vi "Reference Imaging Source.vi"() -> ()   [LabVIEW 2014]
uses:
  <vilib>/userdefined/High Color/IMAQdx.ctl
  <vilib>/vision/driver/IMAQdx.llb/IMAQdx Buffer Number Mode.ctl
  <vilib>/vision/driver/NI_Vision_Acquisition_Software.lvlib
  <resource>/objmgr/imaqdx.rc
panel:
  out "Ref Path":path
  out "Init Message":string
  out "Device Serial Number":string
  out "Success?":bool
  out "error out  - closing camera":errorcluster
  out "Message":string
  out "Warning":bool
  in  "Overwrite?":bool
  in  "Exposure Time":dbl=1.0 min=5e-06 max=5.0 step=1e-05 format="%#_8f"
  out "Buffer Number Out":u32
  in  "Nom Ref":string="ref"
  in  "File Path (for Snap! function)":path
  in  "snap":bool
  in  "Gain (dB)":i64=18 min=34 max=255 step=1
  in  "File to ref":bool
  in  "Ref To File":bool
  in  "End Point 2":cluster{"X":i32, "Y":i32}
  in  "Start Point 2":cluster{"X":i32, "Y":i32}
  in  "End Point 1":cluster{"X":i32, "Y":i32}
  in  "Start Point 1":cluster{"X":i32, "Y":i32}
  out "error out":errorcluster
  in  "error in (no error)":errorcluster
  in  "Rectangle d'encardrement":T1
  in  "ref":bool
  out "Coordonnées":i32[](array[numeric])
  in  "stop":bool
  out "Image":T2(plugin-control)
  in  "Session":T3="cam0"
  # "Références Champs Proches/Champs Lointains"
  # "Utiliser outil OVALE pour effectuer la sélection"
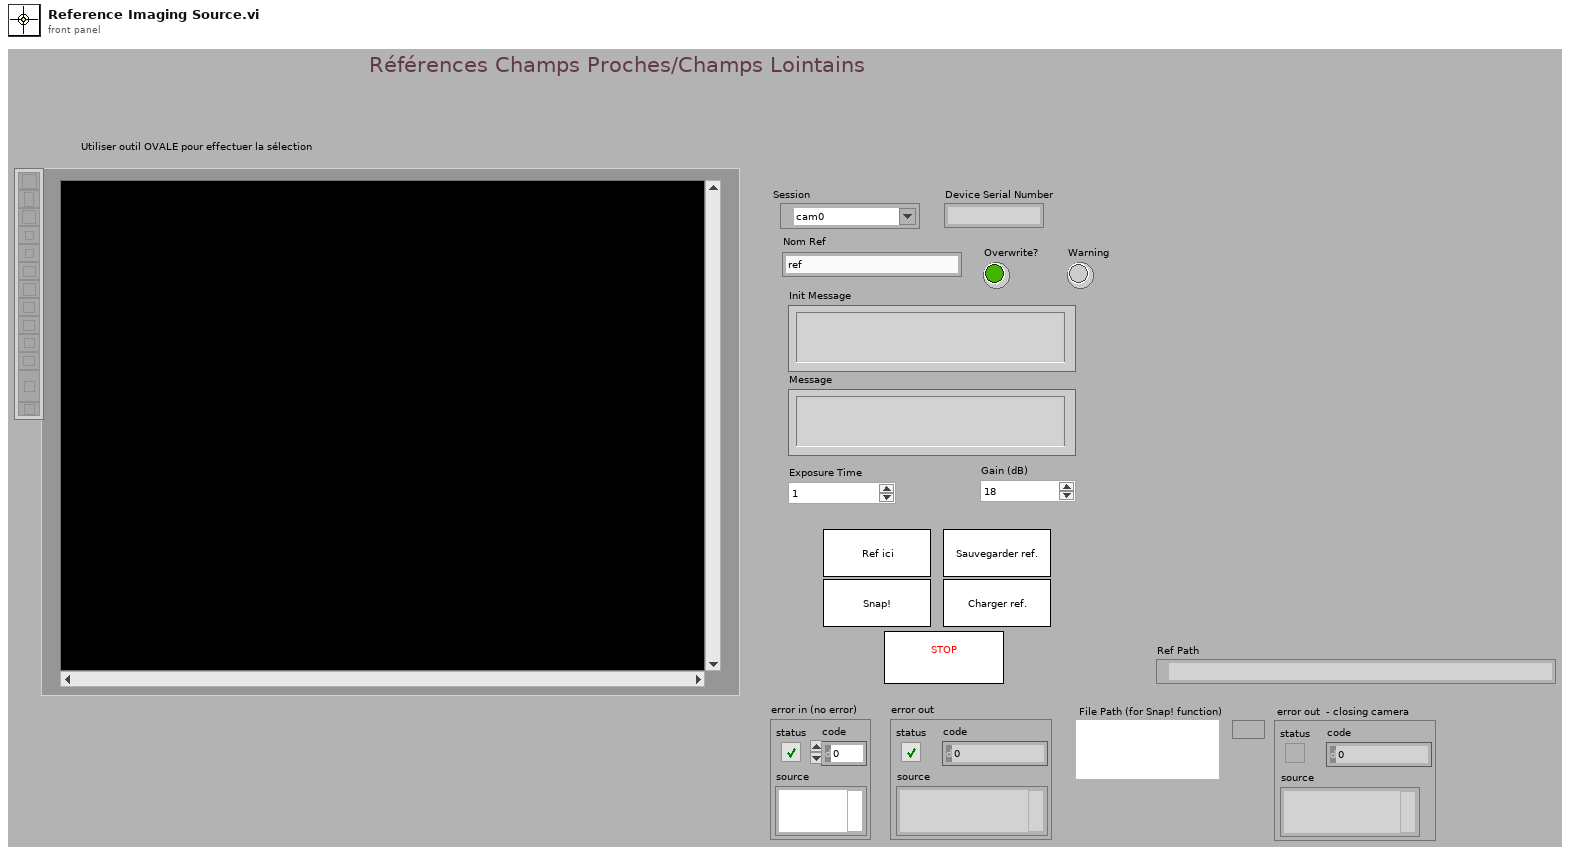
[diagram p1: front panel]
types:
  T1 = cluster{"Left":i32, "Top":i32, "Right":i32, "Bottom":i32}
  T2 = typedef "IMAQ Image.ctl" = refnum<image>
  T3 = typedef "IMAQdx.ctl" = refnum<k21>
  T4 = enum16{"open", "replace", "create", "open or create", "replace or create", "replace or create with confirmation"}
  T5 = typedef "NI_Vision_Acquisition_Software.lvlib/IMAQdx Buffer Number Mode.ctl" = enum32{"Next", "Last", "Buffer Number"}
  T6 = enum8{"Enabled", "Disabled", "Disabled and Grayed Out"}
  T7 = typedef "Image Type" = u32
  T8 = cluster{"Start Point 1":cluster{"X":i32, "Y":i32}, "End Point 1":cluster{"X":i32, "Y":i32}, "Start Point 2":cluster{"X":i32, "Y":i32}, "End Point 2":cluster{"X":i32, "Y":i32}}
  T9 = enum32{"invalid app kind", "Development System", "Run Time System", "Student Edition", "Embedded LabVIEW", "Evaluation", "Custom"}
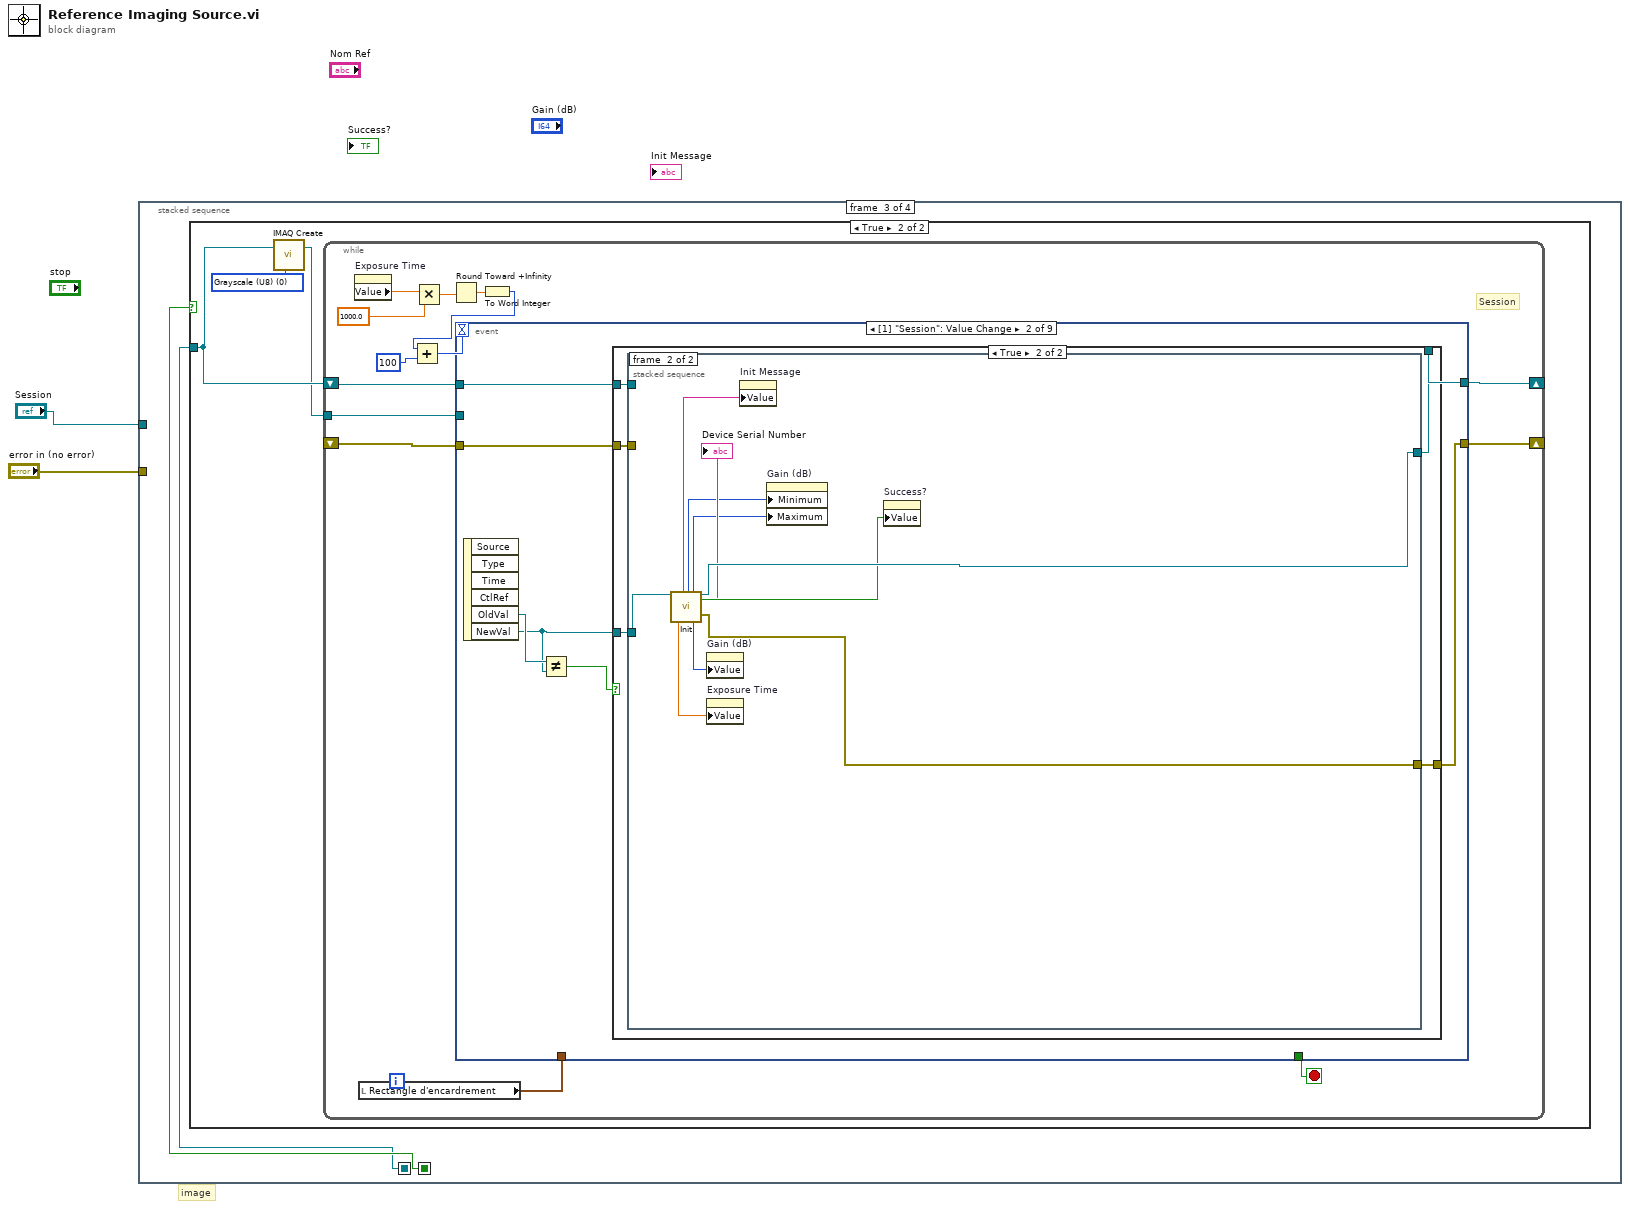
[diagram p0: block diagram]
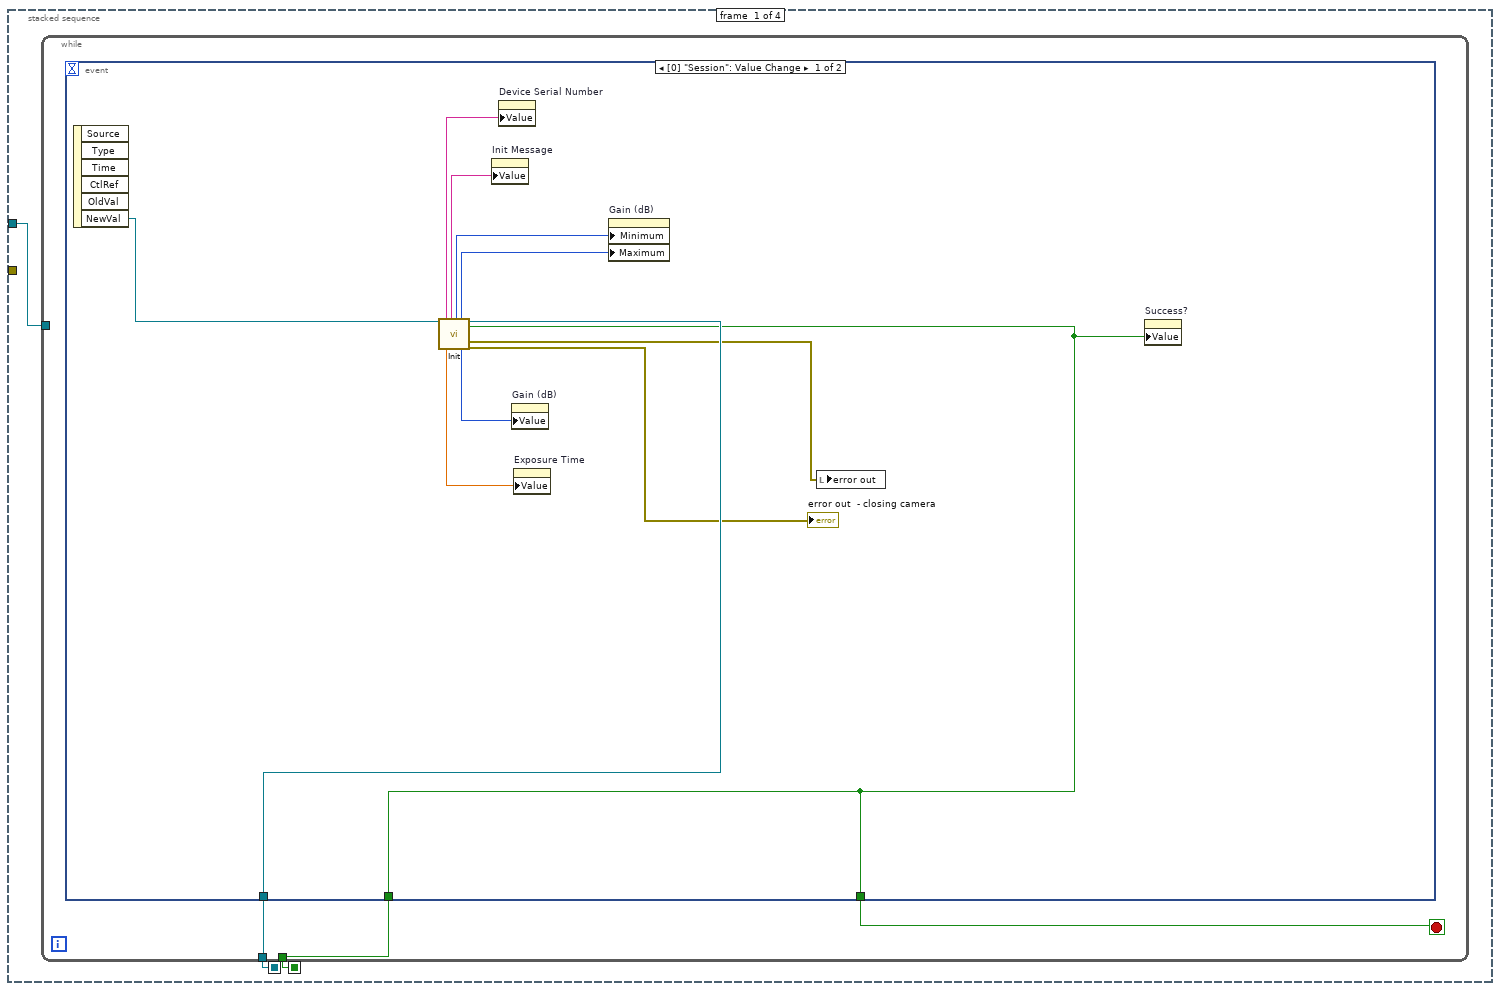
[diagram p2: hidden frame]
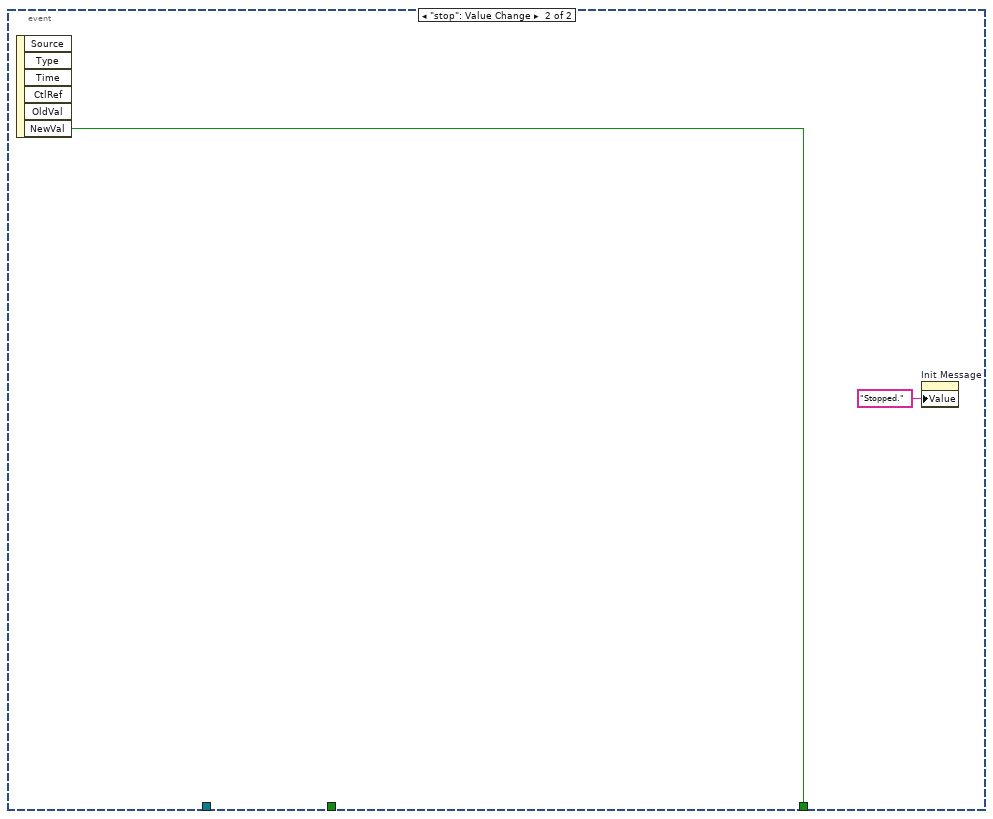
[diagram p3: hidden frame]
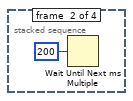
[diagram p4: hidden frame]
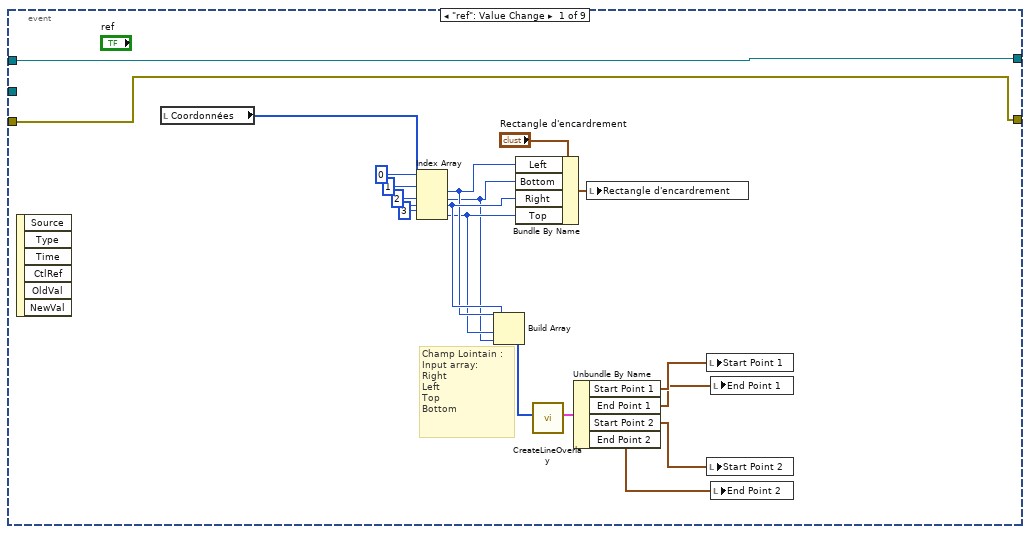
[diagram p6: hidden frame]
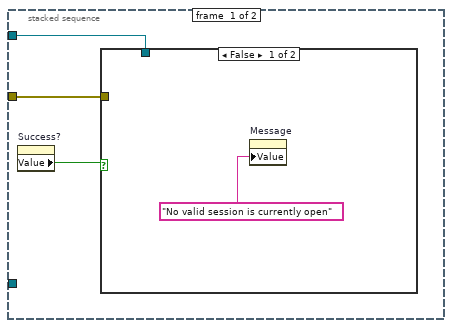
[diagram p8: hidden frame]
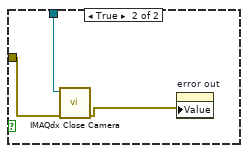
[diagram p9: hidden frame]
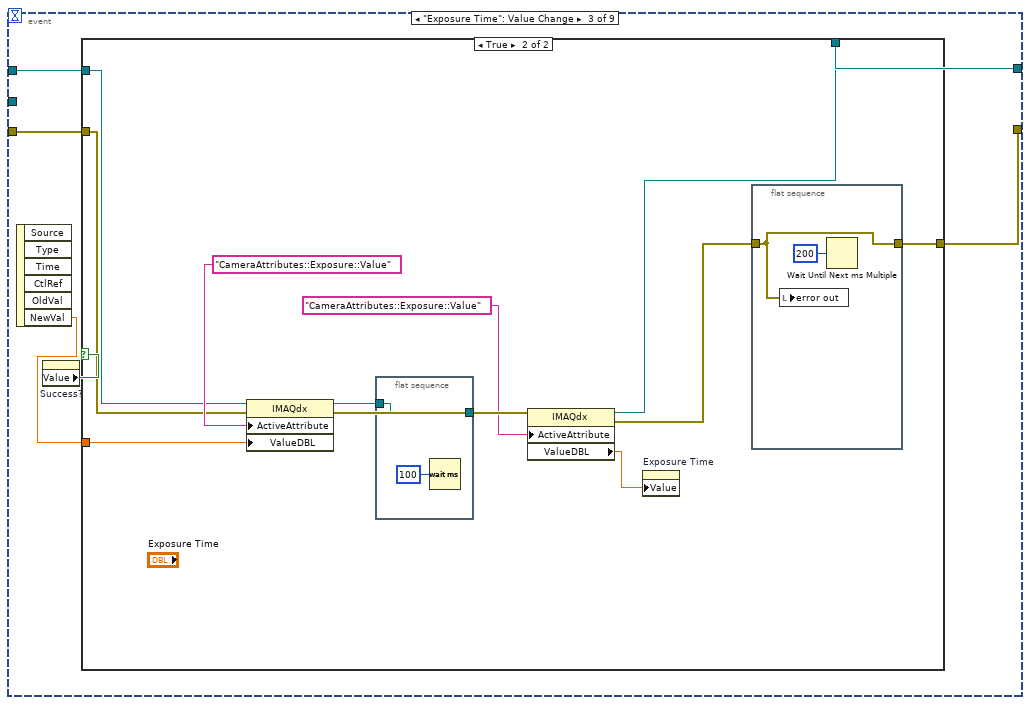
[diagram p10: hidden frame]
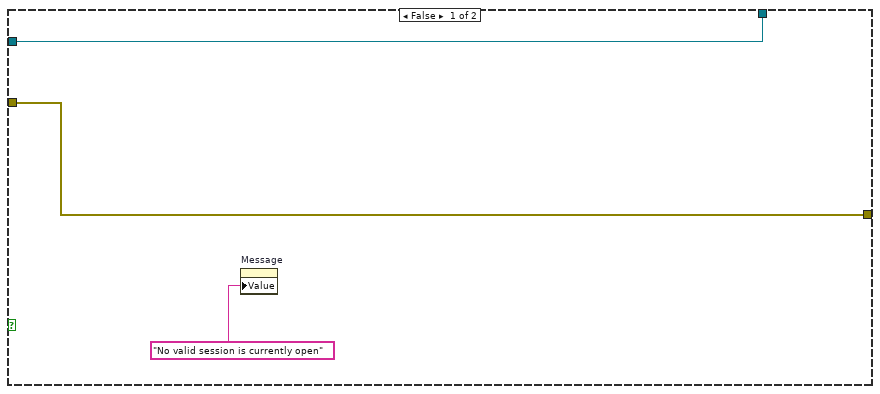
[diagram p11: hidden frame]
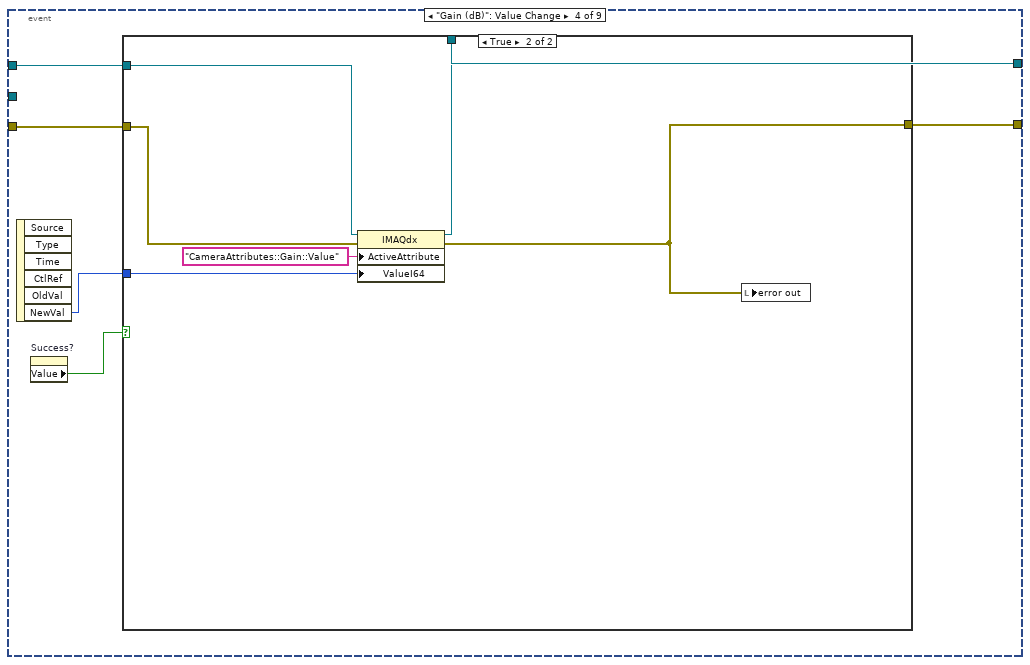
[diagram p12: hidden frame]
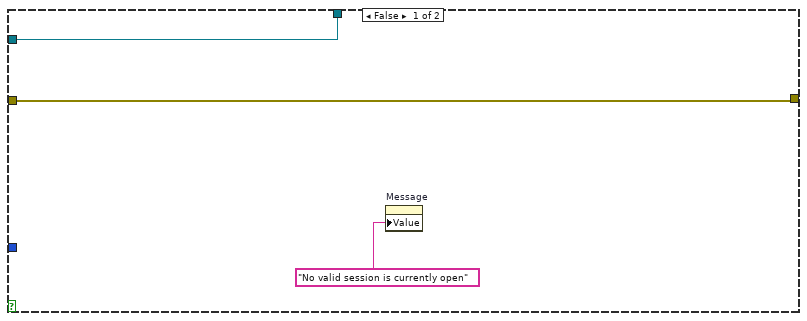
[diagram p13: hidden frame]
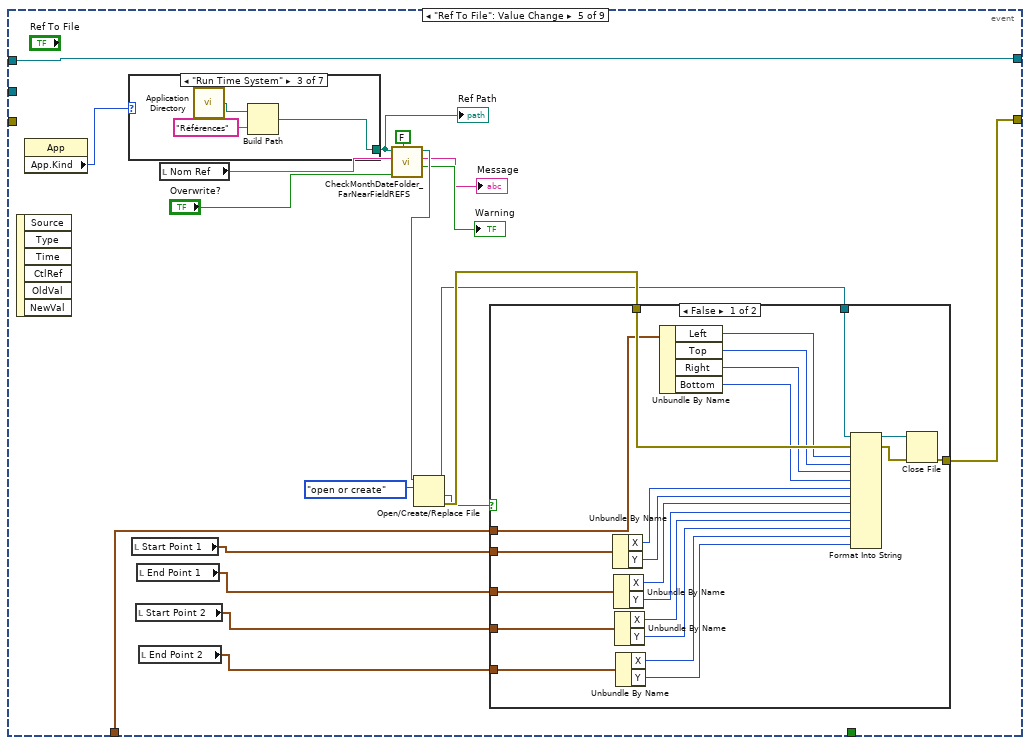
[diagram p14: hidden frame]
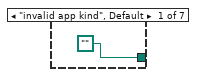
[diagram p15: hidden frame]
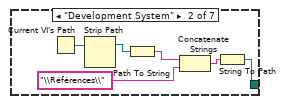
[diagram p16: hidden frame]
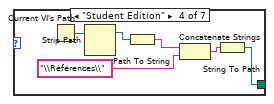
[diagram p17: hidden frame]
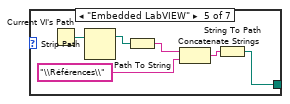
[diagram p18: hidden frame]
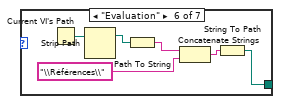
[diagram p19: hidden frame]
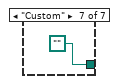
[diagram p20: hidden frame]
diagram:
  # "image"
  n1 = stacked-sequence {
    seq-local: [w4 _ _ _] -> [_ _ w23 _]
    seq-local: [w3 _ _ _] -> [_ _ w24 _]
    tunnel: "Session" -> [w5 _ _ _]
    tunnel: "error in (no error)" -> [_ _ _ _]
    frame #0 {
      n2 = while {
        tunnel: w5 -> [_]
        tunnel: [w7] -> w4
        tunnel: [w6] -> w3
        stop <- w8 stop-if-true
        n3 = event shown="[0] \"Session\": Value Change" {
          selector: _ -> [_ _]
          dyn-events: _ -> [_ _]
          timeout: _ -> [_ _]
          tunnel: [w11 w21] -> w8
          tunnel: [w19 _] -> w7
          tunnel: [w11 _] -> w6
          event Value Change {
            n4 = event-data() -> ("NewVal"=w18:T3)  [unwired: 1 in, 5 out]
            n5 = call "Init.vi"("Session"=w18) -> ("Device Serial Number"=w12:string, "Exposure Time - READ"=w16:dbl, "Message"=w13:string, "Gain Min"=w10:i64, "Gain Max"=w9:i64, "Gain - READ"=w17:i64, "IMAQdx Session OUT"=w19:T3, "Success?"=w11:bool, "error out"=w15:errorcluster, "error out  - closing camera"=→"error out  - closing camera":errorcluster)  [unwired: 9 in]
            n6 = property on="Init Message" class="Str"("Value"=w13) -> ()  [unwired: 2 in, 2 out]
            n7 = property on="Device Serial Number" class="Str"("Value"=w12) -> ()  [unwired: 2 in, 2 out]
            n8 = property on="Gain (dB)" class="DigNum (strict)"("Value"=w17) -> ()  [unwired: 2 in, 2 out]
            n9 = property on="Exposure Time" class="DigNum (strict)"("Value"=w16) -> ()  [unwired: 2 in, 2 out]
            n10 = property on="Gain (dB)" class="DigNum (strict)"("Minimum"=w10, "Maximum"=w9) -> ()  [unwired: 2 in, 2 out]
            n11 = local write "error out"(w15) -> ()
            n12 = property on="Success?" class="Bool (strict)"("Value"=w11) -> ()  [unwired: 2 in, 2 out]
          }
          event "stop": Value Change {
            n13 = event-data() -> ("NewVal"=w21:bool)  [unwired: 1 in, 5 out]
            n14 = property on="Init Message" class="Str"("Value"="Stopped." ("Init Message")) -> ()  [unwired: 2 in, 2 out]
          }
        }
      }
    }
    frame #1 {
      n15 = Wait Until Next ms Multiple(millisecond multiple=u32 200) -> ()  [unwired: 1 out]
    }
    frame #2 {
      n16 = case shown="True" w24 {
        tunnel: w23 -> [_ w26]
        frame False {
        }
        frame True {
          w27 = T7 0 items=["Grayscale (U8)", "Grayscale (I16)", "Grayscale (SGL)", "Complex (CSG)", "RGB (U32)", "HSL (U32)", "RGB (U64)", "Grayscale (U16)"] ("Image Type")
          n17 = call "IMAQ Create"("Image Name"=w26, "Image Type"=w27) -> ("New Image"=w25:T2)  [unwired: 2 in, 2 out]
          n18 = while {
            shift-right: [w39] -> _
            shift-left: _ -> [w40]
            shift-right: [w37] -> _
            shift-left: w26 -> [w38]
            tunnel: w25 -> [w28]
            stop <- w41 stop-if-true
            # "Session"
            n19 = property on="Exposure Time" class="DigNum (strict)"() -> ("Value"=w29:dbl)  [unwired: 2 in, 2 out]
            n20 = local read "Rectangle d'encardrement"() -> (w30:T1)
            n21 = Multiply(x=w29, y=1000.0) -> (x*y=w32:dbl)
            n22 = Round Toward +Infinity(x=w32) -> (ceil(x): smallest int >= x=w34:dbl)
            n23 = To Word Integer(number=w34) -> (16bit integer=w31:i16)
            n24 = Add(x=w31, y=i16 100) -> (x+y=w35:i16)
            n25 = event shown="[1] \"Session\": Value Change" {
              selector: _ -> [_ _ _ _ _ _ _ _ _]
              dyn-events: _ -> [_ _ _ _ _ _ _ _ _]
              timeout: w35 -> [_ _ _ _ _ _ _ _ _]
              tunnel: [_ _ _ _ _ _ _ w264 _] -> w41
              tunnel: w40 -> [w42 w67 w95 w122 _ w213 w248 w265 w278]
              tunnel: [w42 w65 w97 w119 w146 w208 w249 _ w277] -> w39
              tunnel: w38 -> [w43 w64 w96 w121 w134 w207 w247 w266 w276]
              tunnel: [w43 w66 w94 w120 w134 w207 w246 _ w275] -> w37
              tunnel: w30 -> [_ _ _ _ w145 _ _ _ _]
              tunnel: w28 -> [_ _ _ _ _ _ w245 _ w270]
              event "ref": Value Change {
                # "Champ Lointain :\nInput array:\nRight\nLeft\nTop\nBottom"
                n26 = event-data() -> ()  [unwired: 1 in, 6 out]
                n27 = local read "Coordonnées"() -> (w54:i32[])
                n28 = Index Array(array=w54, index #1=0 ("index"), index #2=1 ("index"), index #3=2 ("index"), index #4=3 ("index")) -> (element #1=w47:i32, element #2=w45:i32, element #3=w48:i32, element #4=w46:i32)
                n29 = Build Array(w48, w47, w46, w45) -> (w44:i32[])
                n30 = Bundle By Name(cluster="Rectangle d'encardrement", "Left"=w47, "Bottom"=w45, "Right"=w48, "Top"=w46) -> (w55:T1)
                n31 = call "CreateLineOverlay.vi"("Bounding rectangle"=w44) -> ("Lines"=w53:T8)  [unwired: 8 in, 1 out]
                n32 = Unbundle By Name(w53) -> ("Start Point 1"=w52:cluster{"X":i32, "Y":i32}, "End Point 1"=w51:cluster{"X":i32, "Y":i32}, "Start Point 2"=w50:cluster{"X":i32, "Y":i32}, "End Point 2"=w49:cluster{"X":i32, "Y":i32})
                n33 = local write "Rectangle d'encardrement"(w55) -> ()
                n34 = local write "Start Point 1"(w52) -> ()
                n35 = local write "Start Point 2"(w50) -> ()
                n36 = local write "End Point 1"(w51) -> ()
                n37 = local write "End Point 2"(w49) -> ()
              }
              event Value Change {
                n38 = event-data() -> ("OldVal"=w62:T3, "NewVal"=w61:T3)  [unwired: 1 in, 4 out]
                n39 = Not Equal?(x=w62, y=w61) -> (x != y?=w63:bool)
                n40 = case shown="True" w63 {
                  tunnel: w67 -> [w68 w74]
                  tunnel: w61 -> [w69 w73]
                  tunnel: [w69 w72] -> w66
                  tunnel: [w68 w71] -> w65
                  tunnel: w64 -> [_ w70]
                  frame False {
                  }
                  frame True {
                    n41 = stacked-sequence {
                      tunnel: w74 -> [w77 _]
                      tunnel: w73 -> [_ w91]
                      tunnel: [_ w88] -> w72
                      tunnel: [_ w86] -> w71
                      tunnel: w70 -> [w76 _]
                      frame #0 {
                        n42 = property on="Success?" class="Bool (strict)"() -> ("Value"=w75:bool)  [unwired: 2 in, 2 out]
                        n43 = case shown="False" w75 {
                          tunnel: w77 -> [_ w81]
                          tunnel: w76 -> [_ w79]
                          frame False {
                            n44 = property on="Message" class="Str"("Value"="No valid session is currently open" ("Message")) -> ()  [unwired: 2 in, 2 out]
                          }
                          frame True {
                            n45 = call <vilib>:"IMAQdx Close Camera.vi"("error in"=w81, "Session In"=w79) -> ("error out"=w80:errorcluster)  [unwired: 9 in]
                            n46 = property on="error out" class="Clust (strict)"("Value"=w80) -> ()  [unwired: 2 in, 2 out]
                          }
                        }
                      }
                      frame #1 {
                        n47 = call "Init.vi"("Session"=w91) -> ("Device Serial Number"=→"Device Serial Number":string, "Exposure Time - READ"=w89:dbl, "Message"=w84:string, "Gain Min"=w83:i64, "Gain Max"=w82:i64, "Gain - READ"=w90:i64, "IMAQdx Session OUT"=w88:T3, "Success?"=w87:bool, "error out"=w86:errorcluster)  [unwired: 9 in, 1 out]
                        n48 = property on="Gain (dB)" class="DigNum (strict)"("Value"=w90) -> ()  [unwired: 2 in, 2 out]
                        n49 = property on="Exposure Time" class="DigNum (strict)"("Value"=w89) -> ()  [unwired: 2 in, 2 out]
                        n50 = property on="Init Message" class="Str"("Value"=w84) -> ()  [unwired: 2 in, 2 out]
                        n51 = property on="Gain (dB)" class="DigNum (strict)"("Minimum"=w83, "Maximum"=w82) -> ()  [unwired: 2 in, 2 out]
                        n52 = property on="Success?" class="Bool (strict)"("Value"=w87) -> ()  [unwired: 2 in, 2 out]
                      }
                    }
                  }
                }
              }
              event "Exposure Time": Value Change {
                n53 = event-data() -> ("NewVal"=w92:dbl)  [unwired: 1 in, 5 out]
                n54 = property on="Success?" class="Bool (strict)"() -> ("Value"=w93:bool)  [unwired: 2 in, 2 out]
                n55 = case shown="True" w93 {
                  tunnel: [w99 w112] -> w97
                  tunnel: w96 -> [w100 w108]
                  tunnel: w95 -> [w99 w109]
                  tunnel: [w100 w107] -> w94
                  tunnel: w92 -> [_ w101]
                  frame False {
                    n56 = property on="Message" class="Str"("Value"="No valid session is currently open" ("Message")) -> ()  [unwired: 2 in, 2 out]
                  }
                  frame True {
                    n57 = property class="IMAQdx"(reference=w108, error in=w109, "ActiveAttribute"="CameraAttributes::Exposure::Value", "ValueDBL"=w101) -> (reference out=w103:T3, error out=w105:errorcluster)
                    n58 = flat-sequence {
                      tunnel: w103 -> [w114]
                      tunnel: [w114] -> w102
                      frame #0 {
                        n59 = Wait (ms)(milliseconds to wait=u32 100) -> ()  [unwired: 1 out]
                      }
                    }
                    n60 = property class="IMAQdx"(reference=w102, error in=w105, "ActiveAttribute"="CameraAttributes::Exposure::Value") -> (reference out=w107:T3, error out=w111:errorcluster, "ValueDBL"=w106:dbl)
                    n61 = property on="Exposure Time" class="DigNum (strict)"("Value"=w106) -> ()  [unwired: 2 in, 2 out]
                    n62 = flat-sequence {
                      tunnel: w111 -> [w115]
                      tunnel: [w115] -> w112
                      frame #0 {
                        n63 = local write "error out"(w115) -> ()
                        n64 = Wait Until Next ms Multiple(millisecond multiple=u32 200) -> ()  [unwired: 1 out]
                      }
                    }
                  }
                }
              }
              event "Gain (dB)": Value Change {
                n65 = event-data() -> ("NewVal"=w117:i64)  [unwired: 1 in, 5 out]
                n66 = property on="Success?" class="Bool (strict)"() -> ("Value"=w118:bool)  [unwired: 2 in, 2 out]
                n67 = case shown="True" w118 {
                  tunnel: w122 -> [w125 w131]
                  tunnel: w121 -> [w124 w129]
                  tunnel: [w124 w128] -> w120
                  tunnel: [w125 w127] -> w119
                  tunnel: w117 -> [_ w126]
                  frame False {
                    n68 = property on="Message" class="Str"("Value"="No valid session is currently open" ("Message")) -> ()  [unwired: 2 in, 2 out]
                  }
                  frame True {
                    n69 = property class="IMAQdx"(reference=w129, error in=w131, "ActiveAttribute"="CameraAttributes::Gain::Value", "ValueI64"=w126) -> (reference out=w128:T3, error out=w127:errorcluster)
                    n70 = local write "error out"(w127) -> ()
                  }
                }
              }
              event "Ref To File": Value Change {
                n71 = event-data() -> ()  [unwired: 1 in, 6 out]
                n72 = property class="App"() -> ("App.Kind"=w133:T9)  [unwired: 2 in, 2 out]
                n73 = case shown="\"Run Time System\"" w133 {
                  tunnel: [path "" w152 w158 w161 w167 w173 path ""] -> w140
                  frame "invalid app kind", Default {
                  }
                  frame "Development System" {
                    n74 = Current VI's Path() -> (path=w157:path)
                    n75 = Strip Path(path=w157) -> (stripped path=w156:path)  [unwired: 1 out]
                    n76 = Path To String(path=w156) -> (string=w155:string)
                    n77 = Concatenate Strings(w155, "\\Références\\") -> (w153:string)
                    n78 = String To Path(string=w153) -> (path=w152:path)
                  }
                  frame "Run Time System" {
                    n79 = call <vilib>:"Application Directory.vi"() -> ("Application Directory"=w160:path)
                    n80 = Build Path(base path=w160, name or relative path="Références") -> (appended path=w158:path)
                  }
                  frame "Student Edition" {
                    n81 = Current VI's Path() -> (path=w166:path)
                    n82 = Strip Path(path=w166) -> (stripped path=w165:path)  [unwired: 1 out]
                    n83 = Path To String(path=w165) -> (string=w164:string)
                    n84 = Concatenate Strings(w164, "\\Références\\") -> (w162:string)
                    n85 = String To Path(string=w162) -> (path=w161:path)
                  }
                  frame "Embedded LabVIEW" {
                    n86 = Current VI's Path() -> (path=w172:path)
                    n87 = Strip Path(path=w172) -> (stripped path=w171:path)  [unwired: 1 out]
                    n88 = Path To String(path=w171) -> (string=w170:string)
                    n89 = Concatenate Strings(w170, "\\Références\\") -> (w168:string)
                    n90 = String To Path(string=w168) -> (path=w167:path)
                  }
                  frame "Evaluation" {
                    n91 = Current VI's Path() -> (path=w178:path)
                    n92 = Strip Path(path=w178) -> (stripped path=w177:path)  [unwired: 1 out]
                    n93 = Path To String(path=w177) -> (string=w176:string)
                    n94 = Concatenate Strings(w176, "\\Références\\") -> (w174:string)
                    n95 = String To Path(string=w174) -> (path=w173:path)
                  }
                  frame "Custom" {
                  }
                }
                "Ref Path" <- w140
                n96 = local read "Start Point 1"() -> (w144:cluster{"X":i32, "Y":i32})
                n97 = local read "Start Point 2"() -> (w142:cluster{"X":i32, "Y":i32})
                n98 = local read "End Point 1"() -> (w143:cluster{"X":i32, "Y":i32})
                n99 = local read "End Point 2"() -> (w141:cluster{"X":i32, "Y":i32})
                n100 = local read "Nom Ref"() -> (w139:string)
                n101 = call "CheckMonthDateFolder_FarNearFieldREFS.vi"("Folder Path Control"=w140, "File Name"=w139, "Overwrite?"="Overwrite?", "Automatic date folder nesting?"=FALSE) -> ("File Path"=w137:path, "Message"=→"Message":string, "Warning"=→"Warning":bool)  [unwired: 4 in]
                n102 = Open/Create/Replace File(file path (use dialog)=w137, operation (0:open)=T4."open or create") -> (refnum out=w148:refnum<file>, cancelled=w147:bool, error out=w149:errorcluster)  [unwired: 4 in]
                n103 = case shown="False" w147 {
                  tunnel: w149 -> [w201 w206]
                  tunnel: w148 -> [w199 _]
                  tunnel: [w185 w202] -> w146
                  tunnel: w145 -> [w184 _]
                  tunnel: w144 -> [w183 _]
                  tunnel: w143 -> [w182 _]
                  tunnel: w142 -> [w181 _]
                  tunnel: w141 -> [w180 _]
                  frame False {
                    n104 = Unbundle By Name(w183) -> ("X"=w195:i32, "Y"=w194:i32)
                    n105 = Unbundle By Name(w182) -> ("X"=w193:i32, "Y"=w192:i32)
                    n106 = Unbundle By Name(w181) -> ("X"=w191:i32, "Y"=w190:i32)
                    n107 = Unbundle By Name(w180) -> ("X"=w189:i32, "Y"=w188:i32)
                    n108 = Unbundle By Name(w184) -> ("Left"=w200:i32, "Top"=w198:i32, "Right"=w197:i32, "Bottom"=w196:i32)
                    n109 = Format Into String(initial string=w199, error in=w201, w200, w198, w197, w196, w195, w194, w193, w192, w191, w190, w189, w188) -> (resulting string=w187:refnum<file>, error out=w186:errorcluster)  [unwired: 1 in]
                    n110 = Close File(refnum=w187, error in=w186) -> (error out=w185:errorcluster)  [unwired: 1 out]
                  }
                  frame True {
                    n111 = Bundle By Name(cluster=w206, "status"=FALSE, "code"=0, "source"="") -> (w202:errorcluster)
                  }
                }
              }
              event "File to ref": Value Change {
                n112 = event-data() -> ()  [unwired: 1 in, 6 out]
                n113 = Open/Create/Replace File(error in=w213, prompt="Fichier à charger", access (0:read/write)=enum16{"read/write", "read-only", "write-only"}."read-only") -> (refnum out=w210:refnum<file>, cancelled=w209:bool, error out=w212:errorcluster)  [unwired: 3 in]
                n114 = case shown="False" w209 {
                  tunnel: w212 -> [w218 _]
                  tunnel: w210 -> [w241 _]
                  tunnel: [w215 errorcluster {"status"=FALSE, "code"=0, "source"=""} ("error out")] -> w208
                  frame False {
                    n115 = Scan From String("%d %d %d %d %d %d %d %d %d %d %d %d" ("format string"), w241, w218) -> (w217:refnum<file>, w216:errorcluster, output 1=w238:i32, output 2=w237:i32, output 3=w236:i32, output 4=w235:i32, output 5=w233:i32, output 6=w232:i32, output 7=w228:i32, output 8=w227:i32, output 9=w224:i32, output 10=w223:i32, output 11=w220:i32, output 12=w219:i32)  [unwired: 12 in]
                    n116 = local read "Rectangle d'encardrement"() -> (w240:T1)
                    n117 = local read "Start Point 2"() -> (w226:cluster{"X":i32, "Y":i32})
                    n118 = local read "End Point 2"() -> (w222:cluster{"X":i32, "Y":i32})
                    n119 = local read "Start Point 1"() -> (w234:cluster{"X":i32, "Y":i32})
                    n120 = local read "End Point 1"() -> (w230:cluster{"X":i32, "Y":i32})
                    n121 = Bundle By Name(cluster=w234, "X"=w233, "Y"=w232) -> (w231:cluster{"X":i32, "Y":i32})
                    n122 = Bundle By Name(cluster=w230, "X"=w228, "Y"=w227) -> (w229:cluster{"X":i32, "Y":i32})
                    n123 = Bundle By Name(cluster=w240, "Left"=w238, "Top"=w237, "Right"=w236, "Bottom"=w235) -> (w239:T1)
                    n124 = Bundle By Name(cluster=w222, "X"=w220, "Y"=w219) -> (w221:cluster{"X":i32, "Y":i32})
                    n125 = Bundle By Name(cluster=w226, "X"=w224, "Y"=w223) -> (w225:cluster{"X":i32, "Y":i32})
                    n126 = local write "Start Point 1"(w231) -> ()
                    n127 = local write "End Point 1"(w229) -> ()
                    n128 = local write "Start Point 2"(w225) -> ()
                    n129 = local write "End Point 2"(w221) -> ()
                    n130 = local write "Rectangle d'encardrement"(w239) -> ()
                    n131 = Close File(refnum=w217, error in=w216) -> (error out=w215:errorcluster)  [unwired: 1 out]
                  }
                  frame True {
                  }
                }
              }
              event "snap": Value Change {
                n132 = event-data() -> ()  [unwired: 1 in, 6 out]
                n133 = property on="Success?" class="Bool (strict)"() -> ("Value"=w244:bool)  [unwired: 2 in, 2 out]
                n134 = case shown="False" w244 {
                  tunnel: [w250 w261] -> w249
                  tunnel: w248 -> [w250 w259]
                  tunnel: w247 -> [w251 w255]
                  tunnel: [w251 w254] -> w246
                  tunnel: w245 -> [_ w253]
                  frame False {
                    n135 = property on="Message" class="Str"("Value"="No valid session is currently open" ("Message")) -> ()  [unwired: 2 in, 2 out]
                  }
                  frame True {
                    n136 = call <vilib>:"IMAQdx Get Image.vi"("Buffer Number Mode (Next)"=IMAQdx_Buffer_Number_Mode."Buffer Number", "error in"=w259, "Image In"=w253, "Session In"=w255) -> ("error out"=w258:errorcluster, "Image Out"=w257:T2, "Session Out"=w254:T3)  [unwired: 4 in, 1 out]
                    n137 = call-poly "IMAQ Write File 2"("error in (no error)"=w258, "File Path"="File Path (for Snap! function)", "Image"=w257) -> ("error out"=w261:errorcluster)  [unwired: 7 in, 1 out]
                  }
                }
              }
              event "stop": Value Change {
                n138 = event-data() -> ("NewVal"=w264:bool)  [unwired: 1 in, 5 out]
                n139 = call <vilib>:"IMAQdx Close Camera.vi"("error in"=w265, "Session In"=w266) -> ("error out"=→"error out":errorcluster)  [unwired: 9 in]
                n140 = property on="Session" class="IMAQdx (strict)"("DisabledEnum"=T6."Enabled" ("Disabled")) -> ()  [unwired: 2 in, 2 out]
                n141 = property on="Init Message" class="Str"("Value"="Stopped." ("Init Message")) -> ()  [unwired: 2 in, 2 out]
                n142 = property on="Message" class="Str"("Value"="" ("Message")) -> ()  [unwired: 2 in, 2 out]
              }
              event Timeout {
                w271 = 5 items=["None", "Selection Tool", "Point Tool", "Line Tool", "Rectangle Tool", "Oval Tool", "Polygon Tool", "ClosedFreehandTool", "Annulus Tool", "Rotated Rectangle Tool", "Zoom Tool", "Pan Tool", "Polyline Tool", "Freehand Tool"] ("Tool")
                n143 = event-data() -> ()  [unwired: 1 in, 3 out]
                n144 = property on="Success?" class="Bool (strict)"() -> ("Value"=w269:bool)  [unwired: 2 in, 2 out]
                n145 = case shown="True" w269 {
                  tunnel: w278 -> [w280 w302]
                  tunnel: [w280 w301] -> w277
                  tunnel: w276 -> [w281 w300]
                  tunnel: [w281 w299] -> w275
                  tunnel: w270 -> [_ w284]
                  frame False {
                    n146 = property on="Message" class="Str"("Value"="No valid session is currently open" ("Message")) -> ()  [unwired: 2 in, 2 out]
                  }
                  frame True {
                    n147 = property on="Message" class="Str"("Value"="Running..." ("Message")) -> ()  [unwired: 2 in, 2 out]
                    n148 = call <vilib>:"IMAQdx Get Image.vi"("Buffer Number Mode (Next)"=IMAQdx_Buffer_Number_Mode."Buffer Number", "error in"=w302, "Image In"=w284, "Session In"=w300) -> ("error out"=w282:errorcluster, "Buffer Number Out"=→"Buffer Number Out":u32, "Image Out"=w286:T2, "Session Out"=w299:T3)  [unwired: 4 in]
                    n149 = local read "Rectangle d'encardrement"() -> (w296:T1)
                    n150 = call "IMAQ Overlay Oval"("Color"=u32 16716404, "error in (no error)"=w282, "Bounding Rectangle"=w296, "Image"=w286) -> ("error out"=w288:errorcluster, "Image Out"=w294:T2)  [unwired: 6 in]
                    n151 = call "IMAQ Overlay Line"("error in (no error)"=w288, "End Point"="End Point 1", "Start Point"="Start Point 1", "Image"=w294) -> ("error out"=w295:errorcluster, "Image Out"=w293:T2)  [unwired: 6 in]
                    n152 = call "IMAQ Overlay Line"("error in (no error)"=w295, "End Point"="End Point 2", "Start Point"="Start Point 2", "Image"=w293) -> ("error out"=w301:errorcluster, "Image Out"=→"Image":T2)  [unwired: 6 in]
                    n153 = local write "error out"(w301) -> ()
                  }
                }
                n154 = invoke on="Image" class="ImageControl" method="Get Last Event"() -> ("Tool"=w272:i32, "Coordinates"=w273:i32[])  [unwired: 8 in, 6 out]
                n155 = Equal?(x=w271, y=w272) -> (x = y?=w274:bool)
                n156 = case shown="False" w274 {
                  tunnel: w273 -> [_ w303]
                  frame False {
                  }
                  frame True {
                    "Coordonnées" <- w303
                  }
                }
              }
            }
          }
        }
      }
    }
    frame #3 {
      n157 = property on="stop" class="Bool (strict)"("Value"=FALSE ("stop")) -> ()  [unwired: 2 in, 2 out]
    }
  }
